vi "Calculate Index Array.vi"(8 "error in (no error)":errorcluster, 10 "3D Contour Datatype.lvclass in":refnum<class "3D Contour Datatype.lvclass">, 11 "Plot Representation In":T1) -> (0 "error out":errorcluster, 2 "3D Contour Datatype.lvclass out":refnum<class "3D Contour Datatype.lvclass">, 3 "Plot Representation Out":T1)   [LabVIEW 2020, in "3D Contour Datatype.lvclass"]
uses:
  <vilib>/Math Plots/3D Math Plots/3D Contour/3D Contour Datatype/3D Contour Datatype.lvclass
  <vilib>/Math Plots/3D Math Plots/3D Plot/3D Plot/Typedef/Plot Representation.ctl
  <vilib>/Math Plots/3D Math Plots/3D Plot/3D Plot/Typedef/Range Clusters.ctl
  <vilib>/Math Plots/3D Math Plots/3D Plot/3D Plot/Typedef/Mesh Data.ctl
  <vilib>/Math Plots/3D Math Plots/3D Plot/3D Plot/3D Plot.lvclass
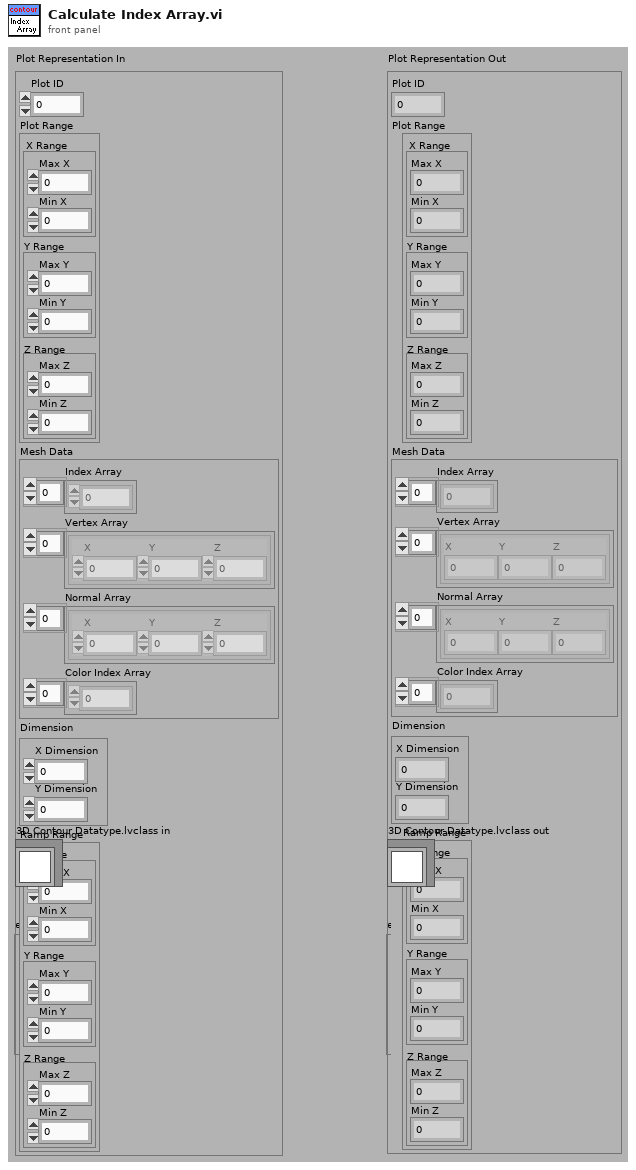
[diagram p1: front panel]
types:
  T1 = typedef "3D Plot.lvclass/Plot Representation.ctl" = cluster{"Plot ID":i32, "Plot Range":T2, "Mesh Data":T3, "Dimension":cluster{"X Dimension":i32, "Y Dimension":i32}, "Ramp Range":T2}
  T2 = typedef "3D Plot.lvclass/Range Clusters.ctl" = cluster{"X Range":cluster{"Max X":sgl, "Min X":sgl}, "Y Range":cluster{"Max Y":sgl, "Min Y":sgl}, "Z Range":cluster{"Max Z":sgl, "Min Z":sgl}}
  T3 = typedef "3D Plot.lvclass/Mesh Data.ctl" = cluster{"Index Array":u32[], "Vertex Array":cluster{"X":sgl, "Y":sgl, "Z":sgl}[], "Normal Array":cluster{"X":sgl, "Y":sgl, "Z":sgl}[], "Color Index Array":i32[]}
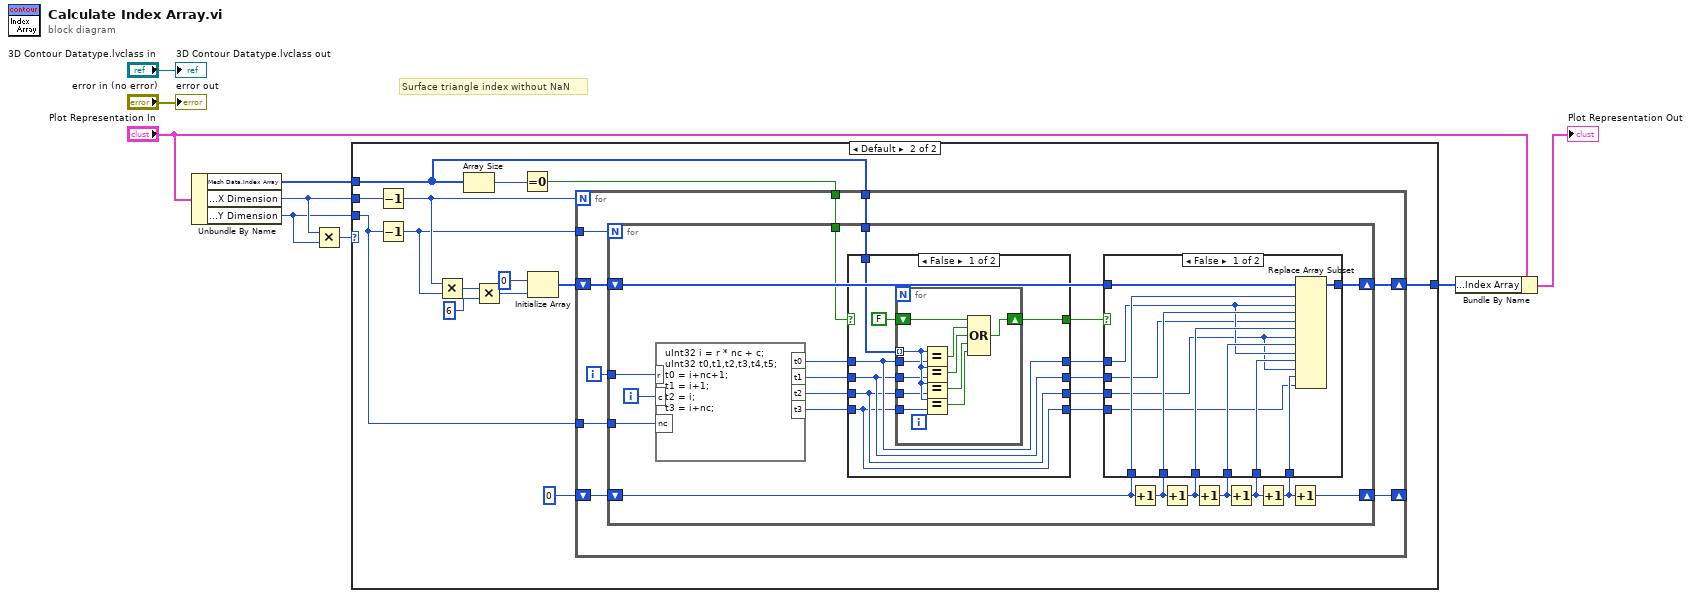
[diagram p0: block diagram]
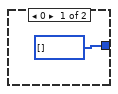
[diagram p2: hidden frame]
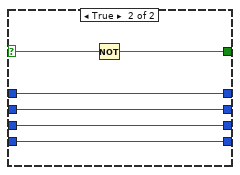
[diagram p4: hidden frame]
diagram:
  # "Surface triangle index without NaN"
  n1 = Unbundle By Name("Plot Representation In") -> ("Mesh Data.Index Array"=w3:u32[], "Dimension.X Dimension"=w2:i32, "Dimension.Y Dimension"=w1:i32)
  n2 = Multiply(x=w2, y=w1) -> (x*y=w5:i32)
  n3 = case shown="Default" w5 {
    tunnel: w2 -> [_ w16]
    tunnel: w1 -> [_ w15]
    tunnel: [u32[] [] w14] -> w4
    tunnel: w3 -> [_ w11]
    frame 0 {
    }
    frame Default {
      n4 = Decrement(x=w16) -> (x-1=w20:i32)
      n5 = Decrement(x=w15) -> (x-1=w19:i32)
      n6 = Multiply(x=w20, y=w19) -> (x*y=w23:i32)
      n7 = Array Size(array=w11) -> (size(s)=w13:i32)
      n8 = Multiply(x=w23, y=6) -> (x*y=w21:i32)
      n9 = Equal To 0?(x=w13) -> (x = 0?=w12:bool)
      n10 = Initialize Array(u32 0, w21) -> (w18:u32[])
      n11 = for {
        N: w20 -> [_]
        shift-right: [w29] -> w14
        shift-left: w18 -> [w33]
        tunnel: w19 -> [w31]
        tunnel: w15 -> [w30]
        shift-right: [w28] -> _
        shift-left: 0 -> [w27]
        tunnel: w12 -> [w26]
        tunnel: w11 -> [w25]
        i -> [w32]
        n12 = for {
          N: w31 -> [_]
          tunnel: w32 -> [w54]
          tunnel: w30 -> [w52]
          shift-right: [w55] -> w29
          shift-left: w33 -> [w56]
          shift-right: [w51] -> w28
          shift-left: w27 -> [w45]
          tunnel: w26 -> [w36]
          tunnel: w25 -> [w35]
          i -> [w53]
          n13 = formula code="uInt32 i = r * nc + c; \nuInt32 t0,t1,t2,t3,t4,t5;\nt0 = i+nc+1; \nt1 = i+1; \nt2 = i; \nt3 = i+nc;"("r"=w54, "nc"=w52, "c"=w53) -> ("t0"=w44:u32, "t1"=w43:u32, "t2"=w42:u32, "t3"=w41:u32)
          n14 = case shown="False" w36 {
            selector: w36 -> [_ w89]
            tunnel: [w73 w93] -> w40
            tunnel: w44 -> [w73 w93]
            tunnel: [w72 w92] -> w39
            tunnel: w43 -> [w72 w92]
            tunnel: [w71 w91] -> w38
            tunnel: w42 -> [w71 w91]
            tunnel: [w70 w90] -> w37
            tunnel: w41 -> [w70 w90]
            tunnel: w35 -> [w76 _]
            tunnel: [w74 w88] -> w34
            frame False {
              n15 = for {
                tunnel: w76 -> [w87] mode=indexing
                tunnel: w73 -> [w86]
                tunnel: w72 -> [w85]
                tunnel: w71 -> [w84]
                tunnel: w70 -> [w83]
                shift-right: [w78] -> w74
                shift-left: FALSE -> [w77]
                n16 = Equal?(x=w87, y=w86) -> (x = y?=w82:bool)
                n17 = Equal?(x=w87, y=w85) -> (x = y?=w81:bool)
                n18 = Equal?(x=w87, y=w84) -> (x = y?=w80:bool)
                n19 = Equal?(x=w87, y=w83) -> (x = y?=w79:bool)
                n20 = Compound Arithmetic op=OR(w77, w82, w81, w80, w79) -> (w78:bool)
              }
            }
            frame True {
              n21 = Not(x=w89) -> (.not. x?=w88:bool)
            }
          }
          n22 = Increment(x=w45) -> (x+1=w46:i32)
          n23 = Increment(x=w46) -> (x+1=w47:i32)
          n24 = Increment(x=w47) -> (x+1=w48:i32)
          n25 = Increment(x=w48) -> (x+1=w49:i32)
          n26 = Increment(x=w49) -> (x+1=w50:i32)
          n27 = case shown="False" w34 {
            tunnel: w56 -> [w68 w69]
            tunnel: [w67 w69] -> w55
            tunnel: w50 -> [w66 _]
            tunnel: w49 -> [w65 _]
            tunnel: w48 -> [w64 _]
            tunnel: w47 -> [w63 _]
            tunnel: w46 -> [w62 _]
            tunnel: w45 -> [w61 _]
            tunnel: w40 -> [w60 _]
            tunnel: w39 -> [w59 _]
            tunnel: w38 -> [w58 _]
            tunnel: w37 -> [w57 _]
            frame False {
              n28 = Replace Array Subset(array=w68, new element #1=w60, index #1=w61, new element #2=w59, index #2=w62, new element #3=w58, index #3=w63, new element #4=w60, index #4=w64, new element #5=w58, index #5=w65, new element #6=w57, index #6=w66) -> (w67:u32[])
            }
            frame True {
            }
          }
          n29 = Increment(x=w50) -> (x+1=w51:i32)
        }
      }
    }
  }
  n30 = Bundle By Name(cluster="Plot Representation In", "Mesh Data.Index Array"=w4) -> (→"Plot Representation Out":T1)
  "error out" <- "error in (no error)"
  "3D Contour Datatype.lvclass out" <- "3D Contour Datatype.lvclass in"
